vi "ContextHelp_DrawString.vi"(0 "PictureIn":picture, 1 "Text":string, 2 "text orientation":T2(ring), 3 "rect":T1={"left"=0, "top"=0, "right"=100, "bottom"=100}, 4 "BoarderSize":i32, 6 "desired font(Application)":T4(ring)=enum."Application Font", 7 "text color(black)":u32(colorbox), 8 "[user-specified font]":T3={"Font Name:"="Ariel", "Size"=20, "Strikeout?"=FALSE, "Italic?"=FALSE, "Underline?"=FALSE, "Outline?"=FALSE, "Shadow?"=FALSE, "Bold?"=FALSE}, 9 "BG color(transparent)":u32(colorbox)=16777216, 10 "BorderColor":u32(colorbox), 11 "H_Offset":i32, 12 "Justify(center)":enum16{"left", "center", "right"}(ring)=enum."center", 13 "V_Offset":i32) -> (14 "PictureOut":picture)   [LabVIEW 2016]
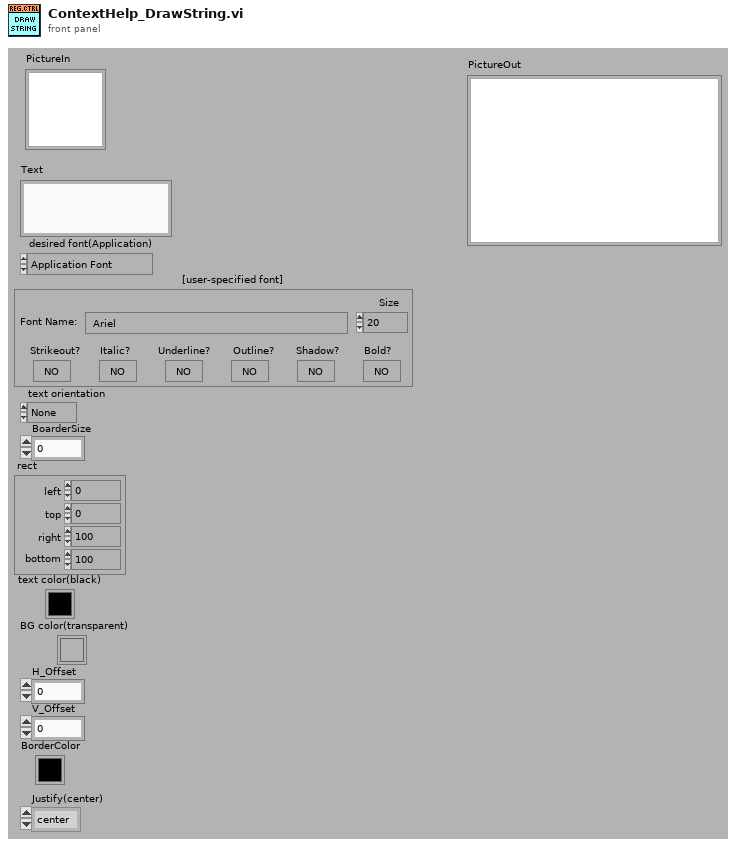
[diagram p1: front panel]
types:
  T1 = cluster{"left":i16, "top":i16, "right":i16, "bottom":i16}
  T2 = enum16{"None", "Stacked", "Clockwise", "Counterclockwise"}
  T3 = cluster{"Font Name:":string, "Size":i16, "Strikeout?":bool, "Italic?":bool, "Underline?":bool, "Outline?":bool, "Shadow?":bool, "Bold?":bool}
  T4 = enum16{"User-specified Font", "Application Font", "System Font", "Dialog Font"}
  T5 = cluster{"horizontal":enum16{"left", "center", "right"}, "vertical":enum16{"top", "center", "bottom"}}
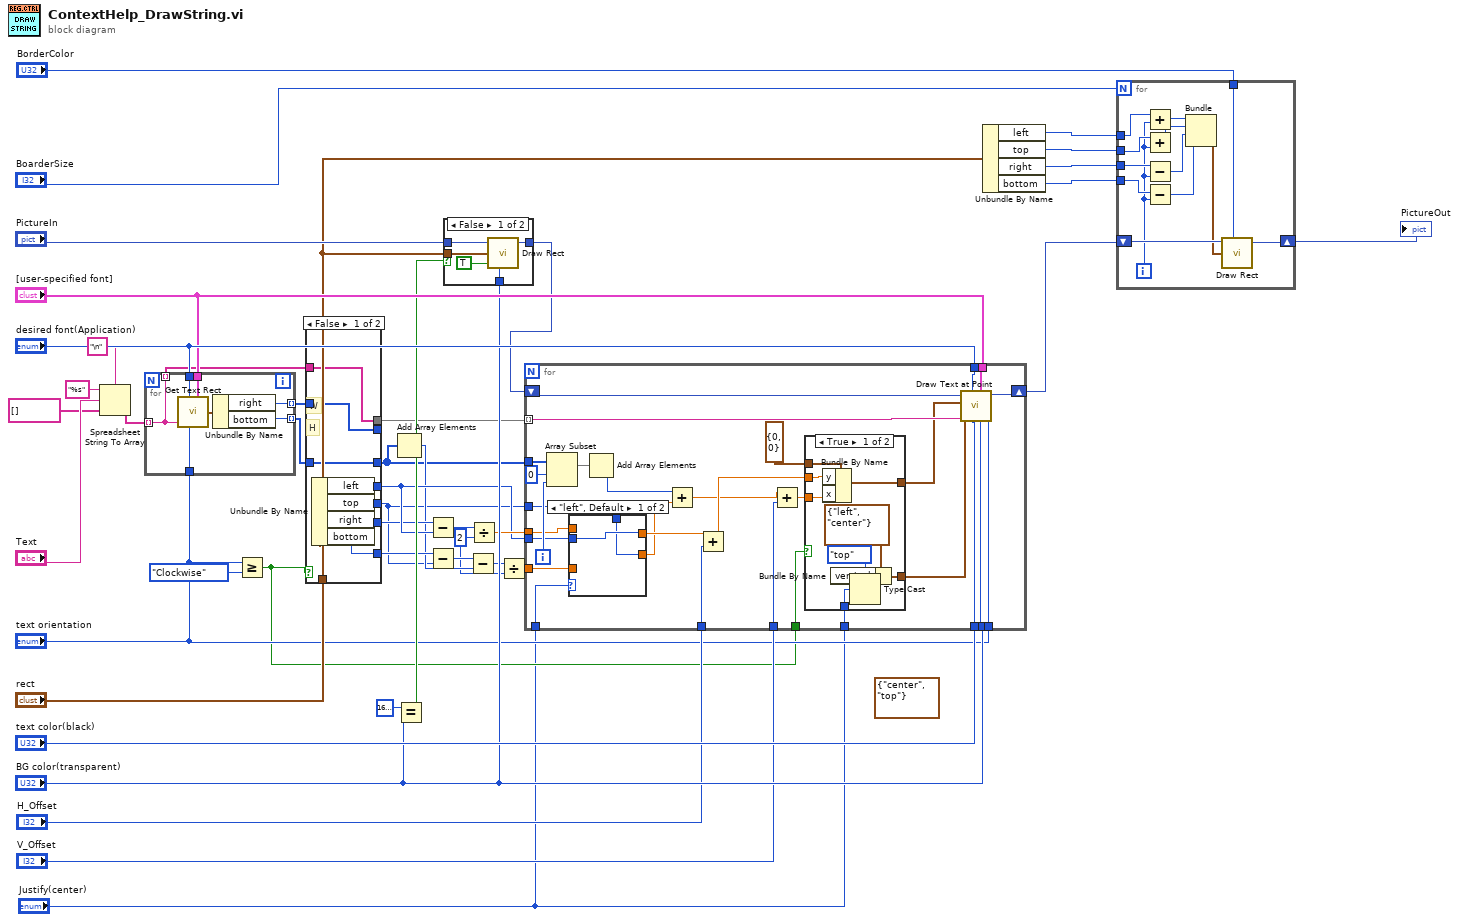
[diagram p0: block diagram]
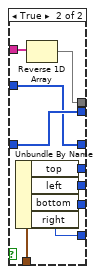
[diagram p2: hidden frame]
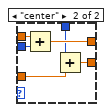
[diagram p4: hidden frame]
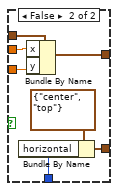
[diagram p5: hidden frame]
diagram:
  (unwired) T5 {"horizontal"=enum."center", "vertical"=enum."top"} ("alignment(left, top)")
  w12 = i16 2 ("y")
  # "H"
  # "W"
  n1 = Spreadsheet String To Array(delimiter (Tab)="\n", format string="%s", spreadsheet string="Text", array type (2D Dbl)=string[] []) -> (array=w37:string[])
  n2 = for {
    tunnel: "desired font(Application)" -> [w51]
    tunnel: "[user-specified font]" -> [w50]
    tunnel: "text orientation" -> [w49]
    tunnel: w37 -> [w45] mode=indexing
    tunnel: [w47] -> w7 mode=indexing
    tunnel: [w46] -> w6 mode=indexing
    tunnel: [w45] -> w3 mode=indexing
    n3 = call <vilib>:"Get Text Rect.vi"("desired font(Application)"=w51, "text"=w45, "text orientation"=w49, "[user-specified font]"=w50) -> ("rect"=w48:T1)  [unwired: 2 in, 3 out]
    n4 = Unbundle By Name(w48) -> ("right"=w47:i16, "bottom"=w46:i16)
  }
  n5 = Greater Or Equal?(x="text orientation", y=T2."Clockwise") -> (x >= y?=w4:bool)
  n6 = case shown="False" w4 {
    tunnel: "rect" -> [w59 w66]
    tunnel: [w58 w62] -> w26
    tunnel: [w57 w65] -> w17
    tunnel: [w56 w63] -> w16
    tunnel: [w55 w64] -> w10
    tunnel: w7 -> [w54 w67]
    tunnel: [w54 w68] -> _
    tunnel: w6 -> [w53 w68]
    tunnel: [w53 w67] -> w5
    tunnel: w3 -> [w52 w61]
    tunnel: [w52 w60] -> w2
    frame False {
      n7 = Unbundle By Name(w59) -> ("left"=w57:i16, "top"=w55:i16, "right"=w56:i16, "bottom"=w58:i16)
    }
    frame True {
      n8 = Unbundle By Name(w66) -> ("top"=w65:i16, "left"=w64:i16, "bottom"=w63:i16, "right"=w62:i16)
      n9 = Reverse 1D Array(array=w61) -> (reversed array=w60:string[])
    }
  }
  n10 = Add Array Elements(numeric array=w5) -> (sum=w14:i16)
  n11 = Equal?(x=u32 16777216 ("BG color(transparent)"), y="BG color(transparent)") -> (x = y?=w30:bool)
  n12 = Subtract(x=w16, y=w17) -> (x-y=w25:i16)
  n13 = Subtract(x=w26, y=w10) -> (x-y=w15:i16)
  n14 = case shown="False" w30 {
    tunnel: "PictureIn" -> [w73 w74]
    tunnel: [w72 w74] -> w20
    tunnel: "rect" -> [w71 _]
    tunnel: "BG color(transparent)" -> [w70 _]
    frame False {
      n15 = call <vilib>:"Draw Rect.vi"("picture"=w73, "rect"=w71, "fill?(F)"=TRUE, "color(black)"=w70) -> ("new picture"=w72:picture)  [unwired: 1 in, 4 out]
    }
    frame True {
    }
  }
  n16 = Subtract(x=w15, y=w14) -> (x-y=w13:i16)
  n17 = Divide(x=w25, y=w12) -> (x/y=w23:dbl)
  n18 = Divide(x=w13, y=w12) -> (x/y=w11:dbl)
  n19 = for {
    tunnel: "desired font(Application)" -> [w96]
    tunnel: "[user-specified font]" -> [w97]
    tunnel: "text color(black)" -> [w93]
    tunnel: "BG color(transparent)" -> [w94]
    shift-right: [w98] -> w19
    shift-left: w20 -> [w99]
    tunnel: w2 -> [w95] mode=indexing
    tunnel: w5 -> [w104]
    tunnel: "V_Offset" -> [w101]
    tunnel: w23 -> [w89]
    tunnel: "H_Offset" -> [w100]
    tunnel: "text orientation" -> [w92]
    tunnel: w17 -> [w85]
    tunnel: w11 -> [w80]
    tunnel: w10 -> [w81]
    tunnel: w4 -> [w78]
    tunnel: "Justify(center)" -> [w76]
    tunnel: "Justify(center)" -> [w75]
    i -> [w103]
    n20 = Array Subset(array=w104, index=0, length=w103) -> (w102:i16[])
    n21 = case shown="\"left\", Default" w75 {
      tunnel: w89 -> [_ w112]
      tunnel: [w106 w111] -> w86
      tunnel: w85 -> [w106 w110]
      tunnel: w81 -> [w105 w109]
      tunnel: w80 -> [_ w108]
      tunnel: [w105 w107] -> w79
      frame "left", Default {
      }
      frame "center" {
        n22 = Add(x=w112, y=w110) -> (x+y=w111:dbl)
        n23 = Add(x=w109, y=w108) -> (x+y=w107:dbl)
      }
    }
    n24 = Add Array Elements(numeric array=w102) -> (sum=w83:i16)
    n25 = Add(x=w83, y=w79) -> (x+y=w82:dbl)
    n26 = Add(x=w86, y=w100) -> (x+y=w88:dbl)
    n27 = Add(x=w82, y=w101) -> (x+y=w84:dbl)
    n28 = case shown="True" w78 {
      tunnel: cluster{"x":i16, "y":i16} {"x"=0, "y"=0} ("origin") -> [w121 w128]
      tunnel: [w120 w127] -> w90
      tunnel: w88 -> [w119 w126]
      tunnel: w84 -> [w118 w125]
      tunnel: [w116 w123] -> w77
      tunnel: w76 -> [w115 w122]
      frame True {
        n29 = Bundle By Name(cluster=w121, "y"=w119, "x"=w118) -> (w120:cluster{"x":i16, "y":i16})
        n30 = Type Cast(type=enum16{"top", "center", "bottom"}."top" ("vertical"), x=w115) -> (*(type *) &x=w113:enum16{"top", "center", "bottom"})
        n31 = Bundle By Name(cluster=T5 {"horizontal"=enum."left", "vertical"=enum."center"} ("alignment(left, top)"), "vertical"=w113) -> (w116:T5)
      }
      frame False {
        n32 = Bundle By Name(cluster=T5 {"horizontal"=enum."center", "vertical"=enum."top"} ("alignment(left, top)"), "horizontal"=w122) -> (w123:T5)
        n33 = Bundle By Name(cluster=w128, "x"=w126, "y"=w125) -> (w127:cluster{"x":i16, "y":i16})
      }
    }
    n34 = call <vilib>:"Draw Text at Point.vi"("text orientation"=w92, "BG color(transparent)"=w94, "[user-specified font]"=w97, "text color(black)"=w93, "desired font(Application)"=w96, "text"=w95, "alignment(left, top)"=w77, "origin"=w90, "picture"=w99) -> ("new picture"=w98:picture)  [unwired: 2 out]
  }
  n35 = Unbundle By Name("rect") -> ("left"=w36:i16, "top"=w35:i16, "right"=w34:i16, "bottom"=w33:i16)
  n36 = for {
    N: "BoarderSize" -> [_]
    shift-right: [w140] -> w18
    shift-left: w19 -> [w141]
    tunnel: w36 -> [w139]
    tunnel: w35 -> [w138]
    tunnel: w34 -> [w137]
    tunnel: w33 -> [w136]
    tunnel: "BorderColor" -> [w134]
    i -> [w135]
    n37 = Add(x=w139, y=w135) -> (x+y=w133:i32)
    n38 = Add(x=w138, y=w135) -> (x+y=w132:i32)
    n39 = Subtract(x=w137, y=w135) -> (x-y=w131:i32)
    n40 = Subtract(x=w136, y=w135) -> (x-y=w130:i32)
    n41 = Bundle(w133, w132, w131, w130) -> (w129:cluster{i32, i32, i32, i32})  [unwired: 1 out]
    n42 = call <vilib>:"Draw Rect.vi"("picture"=w141, "rect"=w129, "color(black)"=w134) -> ("new picture"=w140:picture)  [unwired: 2 in, 4 out]
  }
  "PictureOut" <- w18
